vi "Read NumericLimit Data.vi"(0 "Evaluation Object":refnum<k7>, 11 "error in (no error)":errorcluster) -> (4 "Evaluation Object Out":refnum<k7>, 6 "NumericLimit":T1, 15 "error out":errorcluster)   [LabVIEW 2019, in "STS_LTRV.lvlib"]
uses:
  STS_LTRV.lvlib
  TypeDefs/NumericLimit Data.ctl
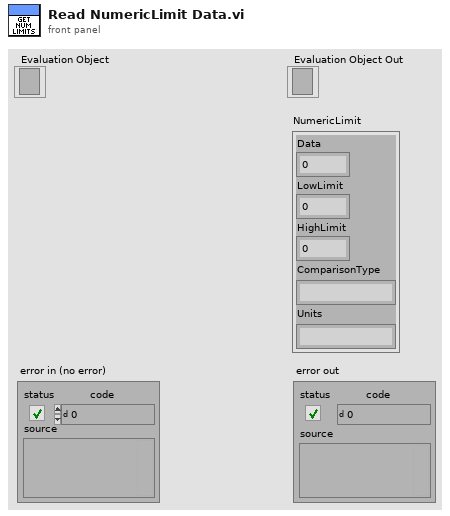
[diagram p1: front panel]
types:
  T1 = typedef "STS_LTRV.lvlib/NumericLimit Data.ctl" = cluster{"Data":dbl, "LowLimit":dbl, "HighLimit":dbl, "ComparisonType":string, "Units":string}
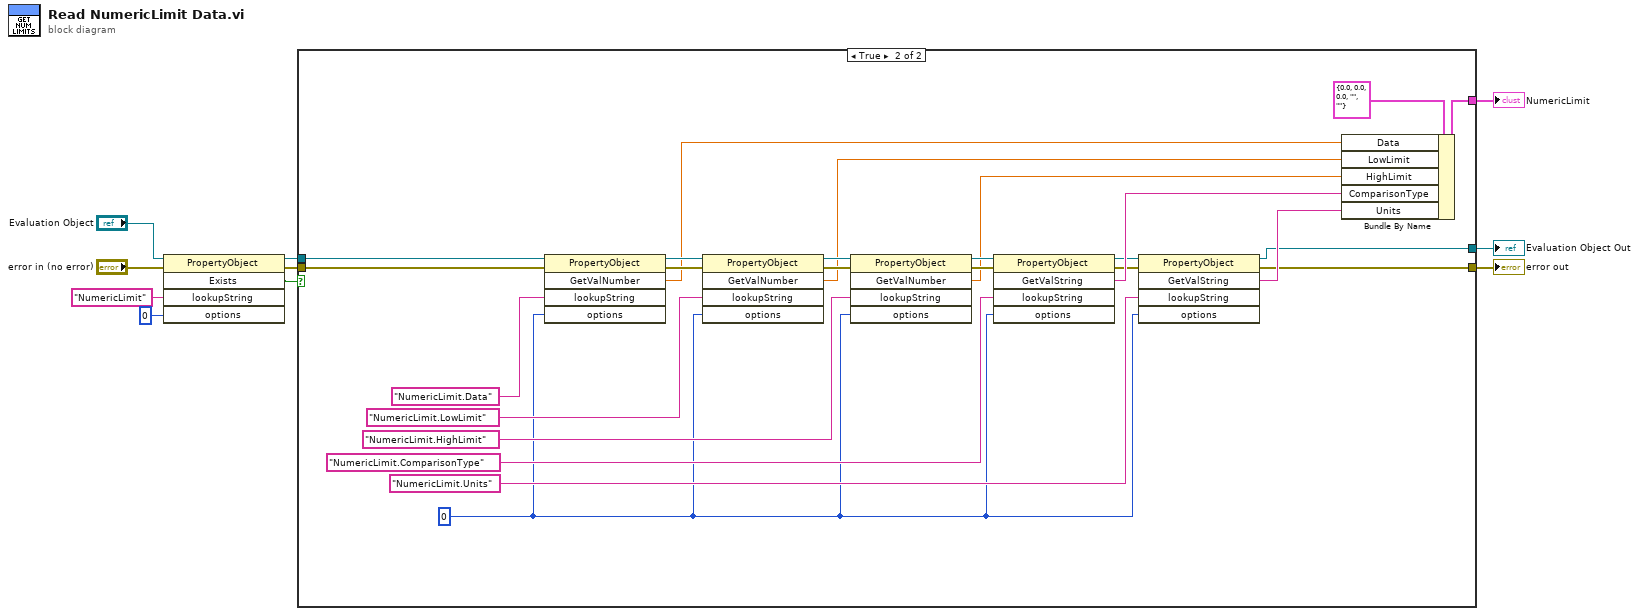
[diagram p0: block diagram]
diagram:
  n1 = invoke class="PropertyObject" method="Exists"(reference="Evaluation Object", error in="error in (no error)", "lookupString"="NumericLimit", "options"=0) -> (reference out=w4:refnum<k7>, error out=w7:errorcluster, "Exists"=w5:bool)  [unwired: 1 in, 2 out]
  n2 = case shown="True" w5 {
    tunnel: w7 -> [w12 w34]
    tunnel: w4 -> [w11 w33]
    tunnel: [w12 w16] -> w3
    tunnel: [_ w15] -> w2
    tunnel: [w11 w13] -> w1
    frame False {
    }
    frame True {
      w14 = 0 ("options")
      n3 = invoke class="PropertyObject" method="GetValNumber"(reference=w33, error in=w34, "lookupString"="NumericLimit.Data", "options"=w14) -> (reference out=w31:refnum<k7>, error out=w32:errorcluster, "GetValNumber"=w25:dbl)  [unwired: 1 in, 2 out]
      n4 = invoke class="PropertyObject" method="GetValNumber"(reference=w31, error in=w32, "lookupString"="NumericLimit.LowLimit", "options"=w14) -> (reference out=w29:refnum<k7>, error out=w30:errorcluster, "GetValNumber"=w24:dbl)  [unwired: 1 in, 2 out]
      n5 = invoke class="PropertyObject" method="GetValNumber"(reference=w29, error in=w30, "lookupString"="NumericLimit.HighLimit", "options"=w14) -> (reference out=w26:refnum<k7>, error out=w27:errorcluster, "GetValNumber"=w23:dbl)  [unwired: 1 in, 2 out]
      n6 = invoke class="PropertyObject" method="GetValString"(reference=w26, error in=w27, "lookupString"="NumericLimit.ComparisonType", "options"=w14) -> (reference out=w20:refnum<k7>, error out=w19:errorcluster, "GetValString"=w22:string)  [unwired: 1 in, 2 out]
      n7 = invoke class="PropertyObject" method="GetValString"(reference=w20, error in=w19, "lookupString"="NumericLimit.Units", "options"=w14) -> (reference out=w13:refnum<k7>, error out=w16:errorcluster, "GetValString"=w17:string)  [unwired: 1 in, 2 out]
      n8 = Bundle By Name(cluster=T1 {"Data"=0.0, "LowLimit"=0.0, "HighLimit"=0.0, "ComparisonType"="", "Units"=""} ("NumericLimit"), "Data"=w25, "LowLimit"=w24, "HighLimit"=w23, "ComparisonType"=w22, "Units"=w17) -> (w15:T1)
    }
  }
  "error out" <- w3
  "NumericLimit" <- w2
  "Evaluation Object Out" <- w1
